vi "HardwareDataNotify.vi"(6 "BPM":cluster{dbl[], "Beam Profile":dbl[]}[](array[cluster]), 8 "Error In":errorcluster, 9 "Hardware Display Data":T1, 10 "ABLE Data Structures":T3, 11 "Hardware Data Structures":T2) -> (0 "Error Out":errorcluster)   [LabVIEW 2012]
uses:
  ABLEDataStructures.ctl
  HardwareDisplayData.ctl
  BPM.ctl
  ExperimentHardwareData.ctl
  ExperimentData.ctl
  AlarmData.ctl
  AlarmDatum.ctl
  HardwareDataStructures.ctl
  PXI6229Data.ctl
  CurrentMeterData.ctl
  HardwareLogData.ctl
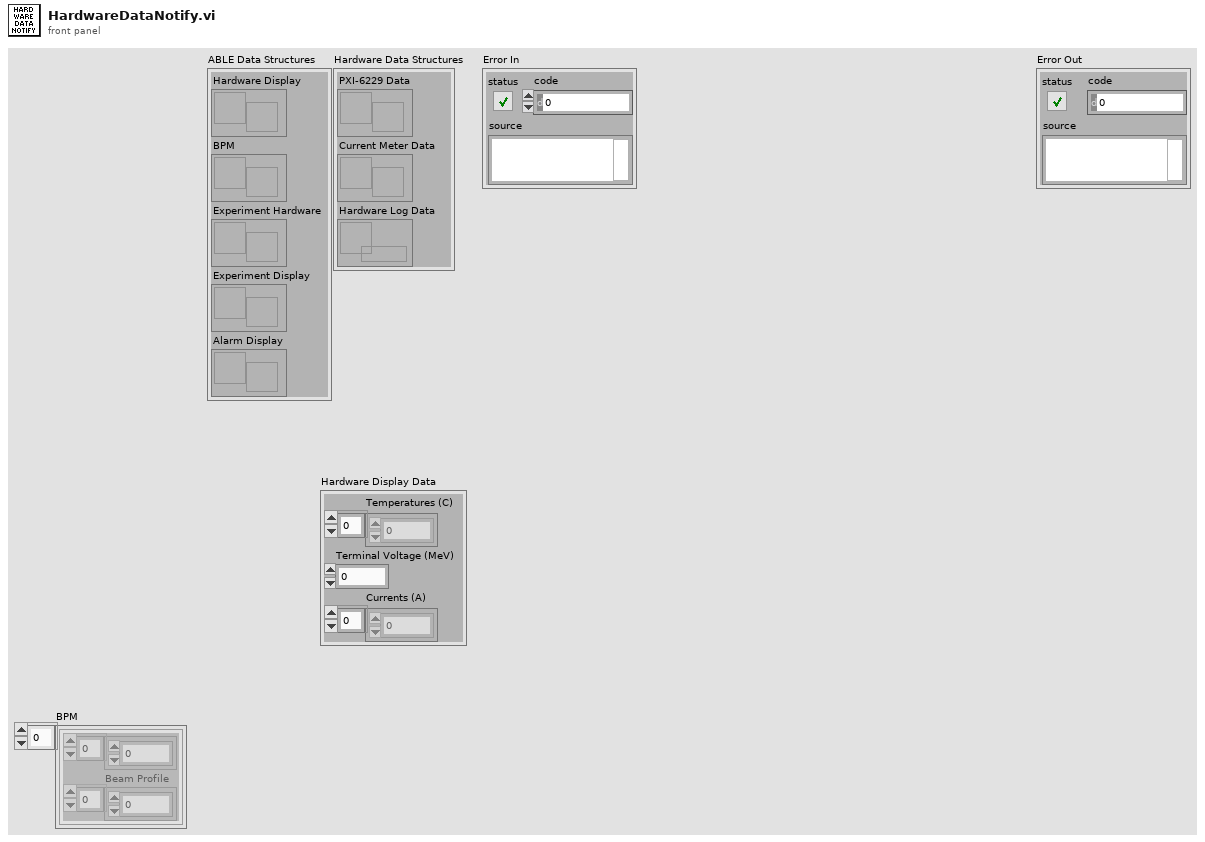
[diagram p1: front panel]
types:
  T1 = typedef "HardwareDisplayData.ctl" = cluster{"Temperatures (C)":dbl[], "Terminal Voltage (MeV)":dbl, "Currents (A)":dbl[]}
  T2 = typedef "HardwareDataStructures.ctl" = cluster{"PXI-6229 Data":refnum<notifier>, "Current Meter Data":refnum<notifier>, "Hardware Log Data":refnum<queue>}
  T3 = typedef "ABLEDataStructures.ctl" = cluster{"Hardware Display":refnum<notifier>, "BPM":refnum<notifier>, "Experiment Hardware":refnum<notifier>, "Experiment Display":refnum<notifier>, "Alarm Display":refnum<notifier>}
  T4 = typedef "ExperimentHardwareData.ctl" = cluster{"Beam Current (A)":dbl, "Terminal Voltage (MeV)":dbl}
  T5 = typedef "HardwareLogData.ctl" = cluster{"Time Stamp":timestamp, "Data":T1}
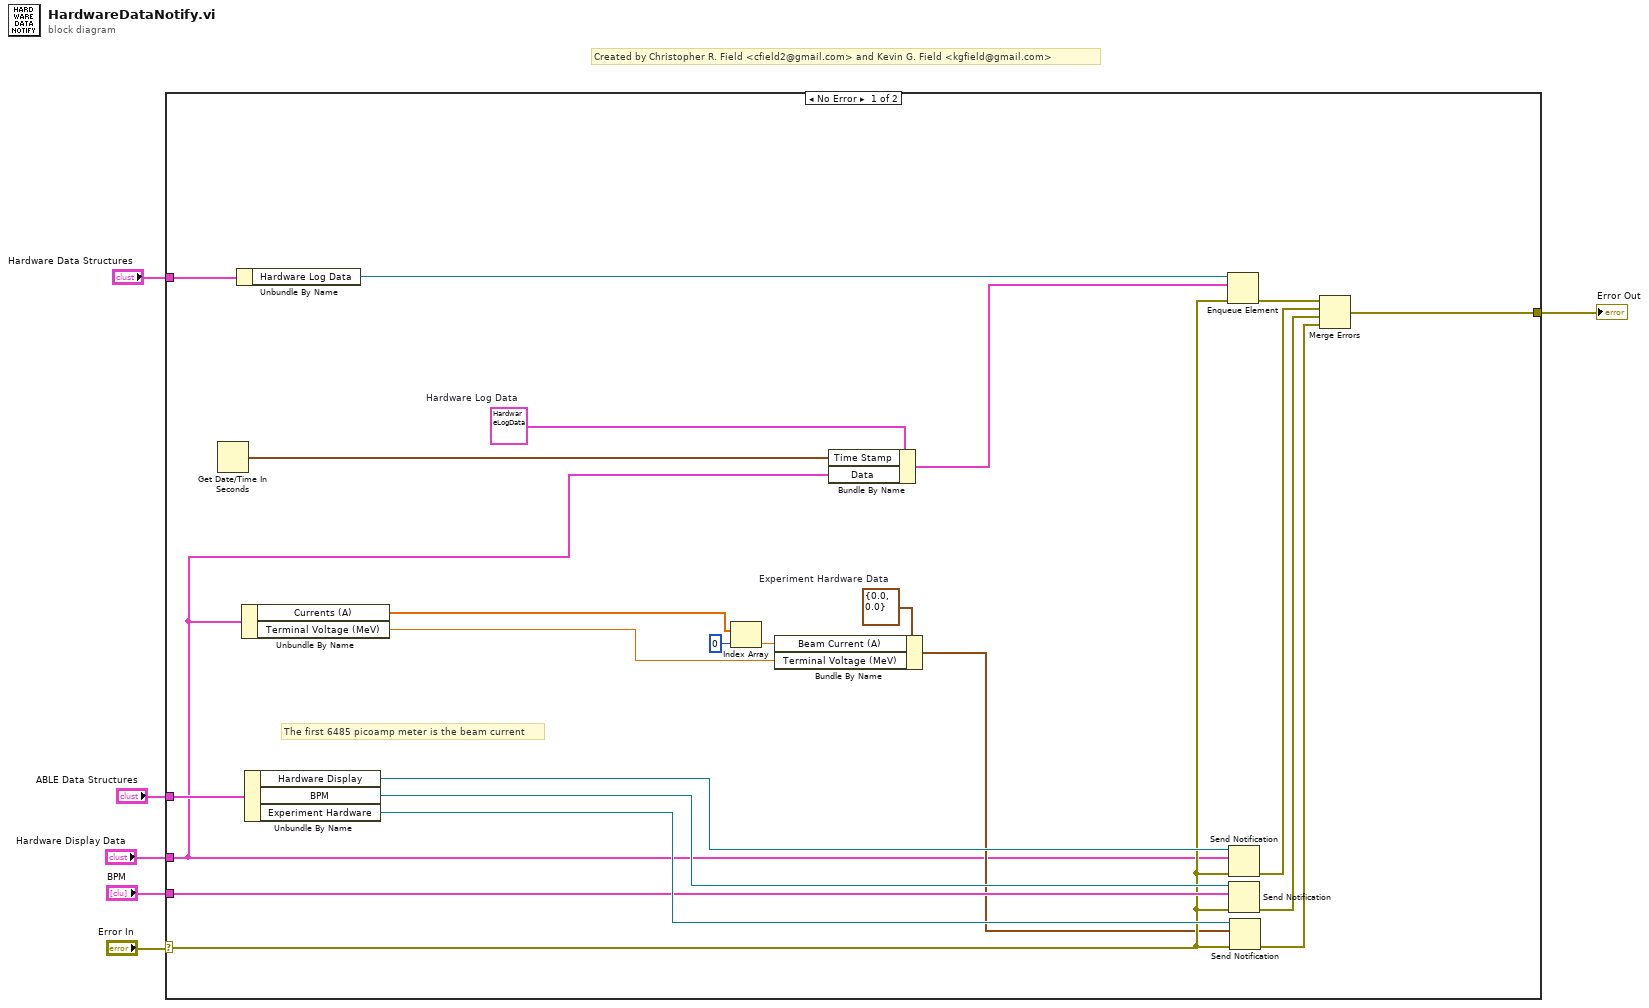
[diagram p0: block diagram]
diagram:
  # "Created by Christopher R. Field <cfield2@gmail.com> and Kevin G. Field <kgfield@gmail.com>"
  n1 = case shown="No Error" "Error In" {
    selector: "Error In" -> [w22 w30]
    tunnel: "ABLE Data Structures" -> [w29 _]
    tunnel: "Hardware Data Structures" -> [w28 _]
    tunnel: "Hardware Display Data" -> [w11 _]
    tunnel: "BPM" -> [w23 _]
    tunnel: [w17 w30] -> w1
    frame No Error {
      w16 = T4 {"Beam Current (A)"=0.0, "Terminal Voltage (MeV)"=0.0}  # Experiment Hardware Data
      w13 = T5 {"Time Stamp"=timestamp(0 s since 1904-01-01), "Data"={"Temperatures (C)"=[], "Terminal Voltage (MeV)"=0.0, "Currents (A)"=[]}}  # Hardware Log Data
      # "The first 6485 picoamp meter is the beam current"
      n2 = Get Date/Time In Seconds() -> (seconds since 1Jan1904=w12:timestamp)
      n3 = Unbundle By Name(w28) -> ("Hardware Log Data"=w24:refnum<queue>)
      n4 = Unbundle By Name(w11) -> ("Currents (A)"=w9:dbl[], "Terminal Voltage (MeV)"=w7:dbl)
      n5 = Unbundle By Name(w29) -> ("Hardware Display"=w27:refnum<notifier>, "BPM"=w26:refnum<notifier>, "Experiment Hardware"=w25:refnum<notifier>)
      n6 = Index Array(array=w9, index=0) -> (element=w8:dbl)
      n7 = Bundle By Name(cluster=w16, "Beam Current (A)"=w8, "Terminal Voltage (MeV)"=w7) -> (w14:T4)
      n8 = Bundle By Name(cluster=w13, "Time Stamp"=w12, "Data"=w11) -> (w10:T5)
      n9 = Enqueue Element(queue=w24, element=w10, error in (no error)=w22) -> (error out=w21:errorcluster)  [unwired: 1 in, 2 out]
      n10 = Send Notification(notification=w11, notifier=w27, error in (no error)=w22) -> (error out=w20:errorcluster)  [unwired: 1 out]
      n11 = Send Notification(notification=w23, notifier=w26, error in (no error)=w22) -> (error out=w19:errorcluster)  [unwired: 1 out]
      n12 = Send Notification(notification=w14, notifier=w25, error in (no error)=w22) -> (error out=w18:errorcluster)  [unwired: 1 out]
      n13 = Merge Errors(w21, w20, w19, w18) -> (w17:errorcluster)
    }
    frame Error {
    }
  }
  "Error Out" <- w1
